vi "FTW-Actor-AddJob-Next.vi"(1 "Add Next in Job Queue":string, 3 "FTW Actor Instance":refnum<class "FTW-Actor-Instance.lvclass">) -> (0 "FTW Actor Instance out":refnum<class "FTW-Actor-Instance.lvclass">)   [LabVIEW 2014, in "FTW-Actor-Instance.lvclass"]
uses:
  FTW-Actor-Instance.lvclass
  FTW-Actor-Instance.lvclass/FTW-Actor-Instance.ctl
  scheduler/FTW-Scheduler.lvclass
panel:
  # "Inputs"
  # "Outputs"
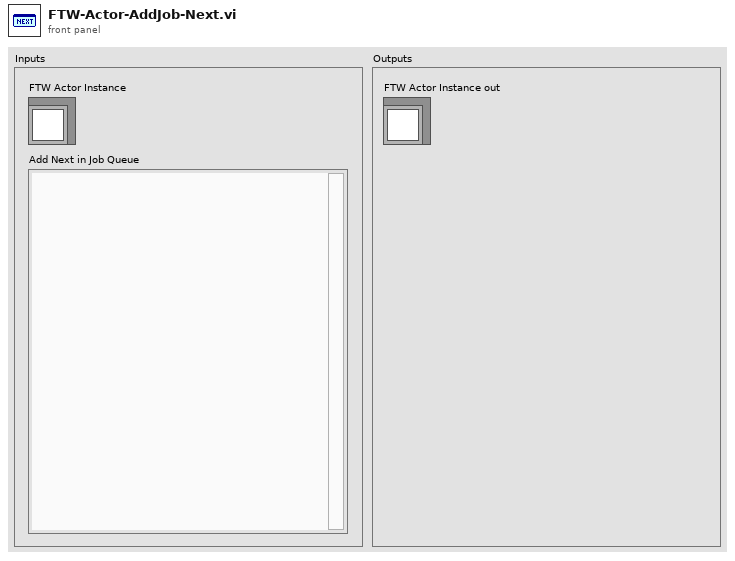
[diagram p1: front panel]
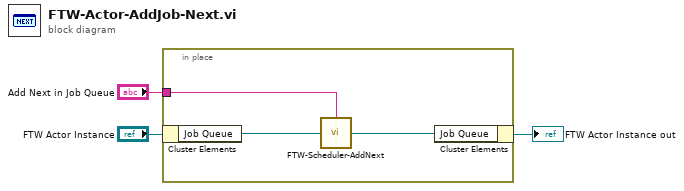
[diagram p0: block diagram]
diagram:
  n1 = in-place {
    in-place-border: "Add Next in Job Queue" -> [w4]
    n2 = in-place-cluster #1("FTW Actor Instance") -> ("Job Queue"=w6:refnum<class "FTW-Scheduler.lvclass">)
    n3 = call "FTW-Scheduler-AddNext.vi"("Add Next in Sequence"=w4, "FTW Job Scheduler"=w6) -> ("FTW Job Scheduler out"=w5:refnum<class "FTW-Scheduler.lvclass">)  [unwired: 2 in]
    n4 = in-place-cluster #1("Job Queue"=w5) -> (→"FTW Actor Instance out":refnum<class "FTW-Actor-Instance.lvclass">)
  }
